vi "_CSMObj-Obtain(OLD).vi"(7 "Allowed Messages(Empty for all)":string[](array[string]), 8 "Error in":errorcluster caption="Error in (no error)", 11 "Requested Name":string) -> (0 "Error out":errorcluster, 3 "CSMQ out":T1={"Core"={"Module Name"="", "Requested Name"="", "Group Name"="", "Mode"=enum."Stand Alone", "User Event"=refnum, "CSM-Data"=refnum, "Allowed Messages"=[]}, "Shared"={"Queue"=refnum, "Status Change Event"=refnum, "TagMap"=refnum, "Mode-Data"=refnum, "Exit Event"=refnum}})   [LabVIEW 2017, in "Communicable State Machine.lvlib"]
uses:
  Communicable State Machine.lvlib
  _CSMObj.ctl
  Priority Queue/Priority Queue.lvclass
  Typedef/_CSM_MODE.ctl
  _CSMObj-Data.ctl
  Typedef/_CSM Status Change Event Data.ctl
  _CSMObj-ModeData.ctl
  Priority Queue/Priority Queue.lvclass/Priority Queue.ctl
  _Shared/CSM Shared.lvlib
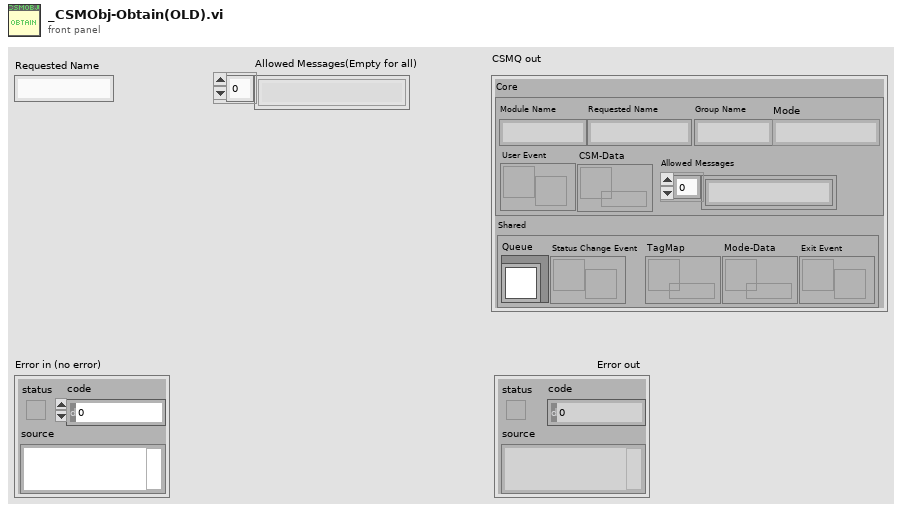
[diagram p1: front panel]
types:
  T1 = typedef "Communicable State Machine.lvlib/_CSMObj.ctl" = cluster{"Core":cluster{"Module Name":string, "Requested Name":string, "Group Name":string, "Mode":T2, "User Event":refnum<user-event>, "CSM-Data":refnum<data-value>, "Allowed Messages":string[]}, "Shared":cluster{"Queue":refnum<class "Priority Queue.lvclass">, "Status Change Event":refnum<user-event>, "TagMap":refnum<data-value>, "Mode-Data":refnum<data-value>, "Exit Event":refnum<user-event>}}
  T2 = typedef "Communicable State Machine.lvlib/_CSM_MODE.ctl" = enum16{"Not Exist", "Stand Alone", "CSM", "Worker", "Worker Agent", "Chain Node", "Chain"}
  T3 = typedef "Communicable State Machine.lvlib/_CSMObj-ModeData.ctl" = cluster{"Share Count":i32, "Messages of Chain Nodes":cluster{"Module Name":string, "Allowed Messages":string[]}[], "Chain Message Mapping Map":variant}
  T4 = typedef "Communicable State Machine.lvlib/_CSMObj-Data.ctl" = cluster{"RemoteMessge?":bool, "error":errorcluster, "InternalRegistryRules":string[], "Return State":string}
  T5 = typedef "Communicable State Machine.lvlib/_CSM_NAME_REQUEST.ctl" = enum16{"Stand Alone CSM Request", "Normal CSM Request", "Agent Request", "Action Worker Request", "Chain Request", "Chain Node Request"}
  T6 = typedef "Communicable State Machine.lvlib/_CSM Status Change Event Data.ctl" = cluster{"ModuleName":string, "Status":string, "Arguments":string}
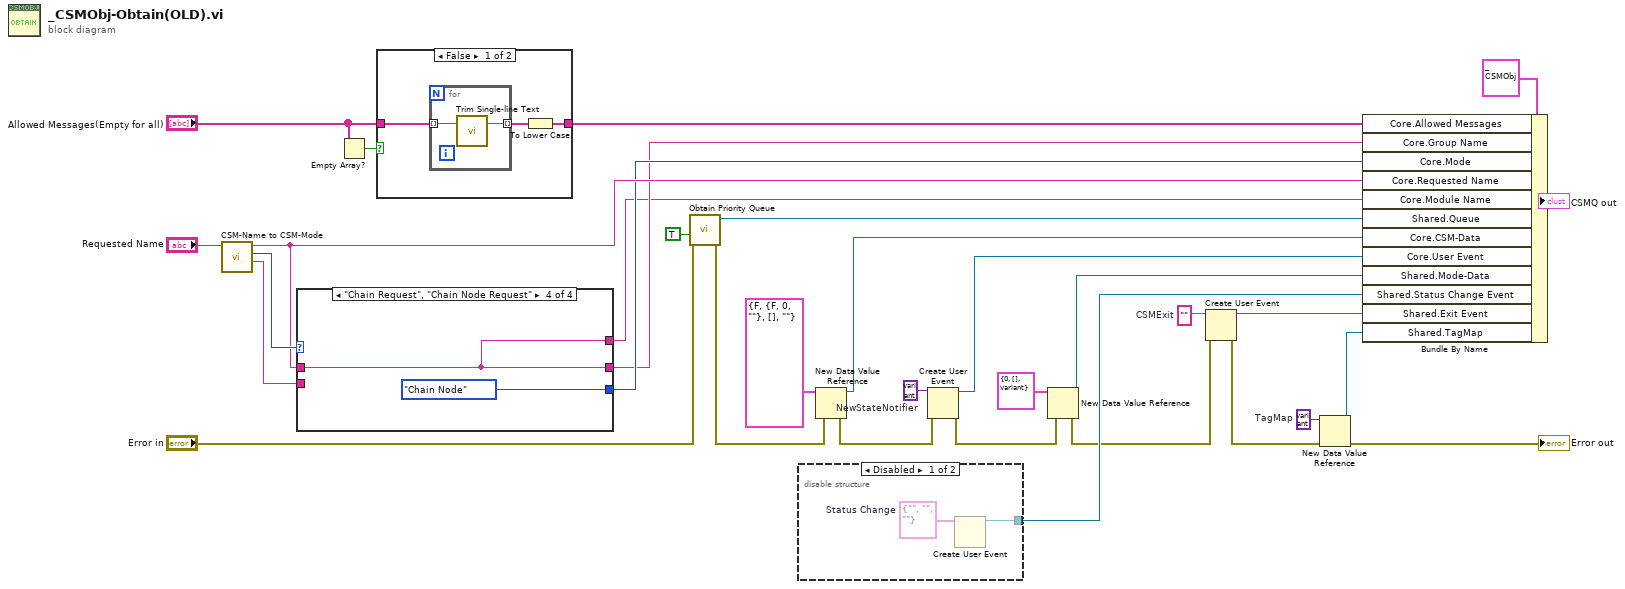
[diagram p0: block diagram]
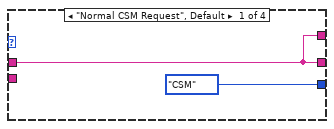
[diagram p2: hidden frame]
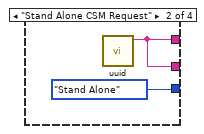
[diagram p3: hidden frame]
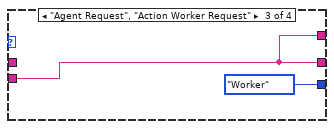
[diagram p4: hidden frame]
diagram:
  w4 = variant  # TagMap
  w7 = ""  # CSMExit
  w29 = variant  # NewStateNotifier
  n1 = call "CSM-Name to CSM-Mode.vi"("String"="Requested Name") -> ("ParentCSM Name"=w18:string, "CSM Mode"=w16:T5, "Requested Name"=w15:string)  [unwired: 8 in]
  n2 = case shown="\"Chain Request\", \"Chain Node Request\"" w16 {
    tunnel: [w33 w35 w37 w39] -> w10
    tunnel: w15 -> [w33 _ _ w39]
    tunnel: w18 -> [_ _ w37 _]
    tunnel: [_CSM_MODE."CSM" ("Mode") _CSM_MODE."Stand Alone" ("Mode") _CSM_MODE."Worker" ("Mode") _CSM_MODE."Chain Node" ("Mode")] -> w14
    tunnel: [w33 w35 w37 w39] -> w9
    frame "Normal CSM Request", Default {
    }
    frame "Stand Alone CSM Request" {
      n3 = call "uuid.vi"() -> ("UUID"=w35:string)  [unwired: 11 in]
    }
    frame "Agent Request", "Action Worker Request" {
    }
    frame "Chain Request", "Chain Node Request" {
    }
  }
  n4 = Empty Array?(array="Allowed Messages(Empty for all)") -> (empty?=w19:bool)
  n5 = case shown="False" w19 {
    tunnel: [w41 w46] -> w21
    tunnel: "Allowed Messages(Empty for all)" -> [w42 w46]
    frame False {
      n6 = for {
        tunnel: [w44] -> w43 mode=indexing
        tunnel: w42 -> [w45] mode=indexing
        n7 = call "Trim Single-line Text.vi"("single-line text"=w45) -> ("trimed text"=w44:string)  [unwired: 2 in]
      }
      n8 = To Lower Case(string=w43) -> (all lower case string=w41:string[])
    }
    frame True {
    }
  }
  n9 = call "Obtain Priority Queue.vi"("error in (no error)"="Error in", "create if not found? (T)"=TRUE) -> ("error out"=w30:errorcluster, "Priority Queue"=w32:refnum<class "Priority Queue.lvclass">)  [unwired: 7 in, 1 out]
  n10 = disable-structure shown="Disabled" {
    disable-tunnel: [w47 _] -> w26
    frame Disabled {
      w48 = T6 {"ModuleName"="", "Status"="", "Arguments"=""}  # Status Change
      n11 = Create User Event(user event datatype=w48) -> (user event=w47:refnum<user-event>)  [unwired: 1 in, 1 out]
    }
    frame Enabled {
    }
  }
  n12 = New Data Value Reference(data value=T4 {"RemoteMessge?"=FALSE, "error"={"status"=FALSE, "code"=0, "source"=""}, "InternalRegistryRules"=[], "Return State"=""} ("CSMObj-Data"), error in=w30) -> (data value reference=w31:refnum<data-value>, error out=w28:errorcluster)
  n13 = Create User Event(user event datatype=w29, error in=w28) -> (user event=w27:refnum<user-event>, error out=w11:errorcluster)
  n14 = New Data Value Reference(data value=T3 {"Share Count"=0, "Messages of Chain Nodes"=[], "Chain Message Mapping Map"=variant} ("CSMObj-Data"), error in=w11) -> (data value reference=w12:refnum<data-value>, error out=w5:errorcluster)
  n15 = Create User Event(user event datatype=w7, error in=w5) -> (user event=w6:refnum<user-event>, error out=w3:errorcluster)
  n16 = New Data Value Reference(data value=w4, error in=w3) -> (data value reference=w1:refnum<data-value>, error out=→"Error out":errorcluster)
  n17 = Bundle By Name(cluster=T1 {"Core"={"Module Name"="", "Requested Name"="", "Group Name"="", "Mode"=enum."Stand Alone", "User Event"=refnum, "CSM-Data"=refnum, "Allowed Messages"=[]}, "Shared"={"Queue"=refnum, "Status Change Event"=refnum, "TagMap"=refnum, "Mode-Data"=refnum, "Exit Event"=refnum}} ("CSMQ in"), "Core.Allowed Messages"=w21, "Core.Group Name"=w10, "Core.Mode"=w14, "Core.Requested Name"=w15, "Core.Module Name"=w9, "Shared.Queue"=w32, "Core.CSM-Data"=w31, "Core.User Event"=w27, "Shared.Mode-Data"=w12, "Shared.Status Change Event"=w26, "Shared.Exit Event"=w6, "Shared.TagMap"=w1) -> (→"CSMQ out":T1)
